vi "List Phone Numbers Opted Out.vi"(8 "error in (no error)":errorcluster, 9 "Region":T1, 11 "AWS Credentials":T2) -> (0 "error out":errorcluster, 3 "Phone Numbers Opted Out":refnum<class "Phone Number.lvclass">[](array[class]))   [LabVIEW 2015, in "NI_AWS_SNS.lvlib" / "Phone Number.lvclass"]
doc: "Returns a list of phone numbers that are opted out, meaning you cannot send SMS messages to them."
uses:
  Phone Number.lvclass
  Core/HTTP Request/AWS Credentials.ctl
  Core/HTTP Request/Region.ctl
  Core/HTTP Request/HTTP Request.lvclass/HTTP Request.ctl
  Core/HTTP Request/Write Credentials.vi
  Core/HTTP Request/Write Region.vi
  Core/HTTP Request/Write Service.vi
  Core/HTTP Request/Write Verify Server.vi
  Core/HTTP Request/HTTP Request.lvclass
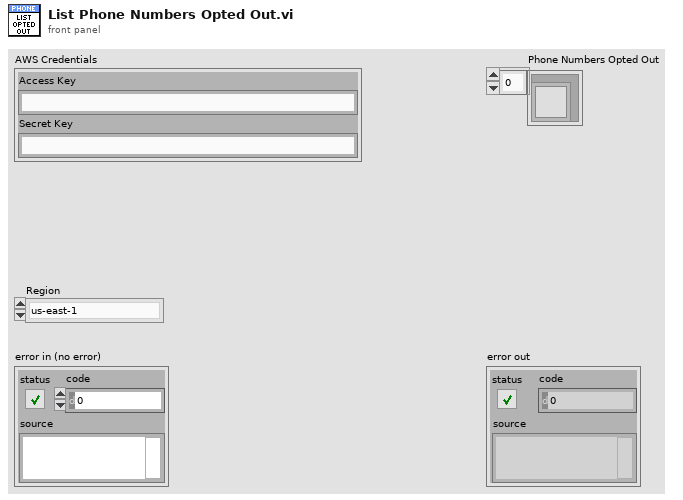
[diagram p1: front panel]
types:
  T1 = typedef "NI_AWS_Core.lvlib/HTTP Request.lvclass/Region.ctl" = enum16{"us-east-1", "us-east-2", "us-west-1", "us-west-2", "ap-northeast-1", "ap-northeast-2", "ap-southeast-1", "ap-southeast-2", "ca-central-1", "eu-central-1", "eu-west-1", "eu-west-2", "sa-east-1"}
  T2 = typedef "NI_AWS_Core.lvlib/HTTP Request.lvclass/AWS Credentials.ctl" = cluster{"Access Key":string, "Secret Key":string}
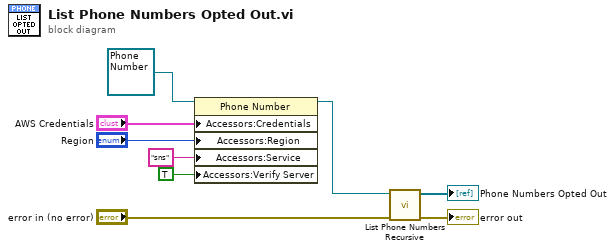
[diagram p0: block diagram]
diagram:
  n1 = property class="Phone Number"(reference=refnum<class "Phone Number.lvclass"> refnum ("NI_AWS_SNS.lvlib:Phone Number.lvclass"), "Accessors:Credentials"="AWS Credentials", "Accessors:Region"="Region", "Accessors:Service"="sns" ("Service"), "Accessors:Verify Server"=TRUE ("Verify Server")) -> (reference out=w4:refnum<class "Phone Number.lvclass">)  [unwired: 1 in, 1 out]
  n2 = call "List Phone Numbers Recursive.vi"("error in (no error)"="error in (no error)", "Phone Number"=w4) -> ("error out"=→"error out":errorcluster, "Phone Numbers Opted Out"=→"Phone Numbers Opted Out":refnum<class "Phone Number.lvclass">[])  [unwired: 8 in]
